vi "Configure Arm Layer Trigger Link.vi"(6 "Enable Output Trigger (F: Disable)":bool, 7 "Arm Output Trigger Line (2: Line2)":i32(ring)=2 items=["Line1"=1, "Line2"=2, "Line3"=3, "Line4"=4, "Line5"=5, "Line6"=6], 8 "error in (no error)":errorcluster, 9 "Arm Input Trigger Line (1: Line1)":i32(ring)=1 items=["Line1"=1, "Line2"=2, "Line3"=3, "Line4"=4, "Line5"=5, "Line6"=6], 10 "Arm Source Bypass (1: Acceptor)":i32(ring)=1 items=["Source", "Acceptor"], 11 "VISA resource name":refnum<visa-resource-name>) -> (0 "error out":errorcluster, 3 "VISA resource name out":refnum<visa-resource-name>)   [LabVIEW 2020, in "Keithley 6517.lvlib"]
doc: "Sets the bypass, input trigger line and output trigger line for the Arm Layer (Arm1) of the trigger model.\n\n<B>Note:</B>\n(1)<B>Models 6517A, 6517B:</B> The trigger model consists of 3 layers, the Arm Layer, the Scan Layer (Arm2), and the Measure Layer (Trigger).\n(2)<B>Model 6514:</B> The trigger model consists of 2 layers: Arm Layer & Measure Layer (Trigger)."
uses:
  <instrlib>/Keithley 6517/Keithley 6517.lvlib
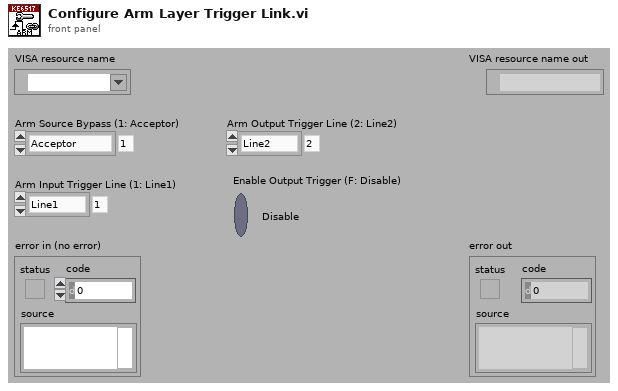
[diagram p1: front panel]
types:
  T1 = typedef "Keithley 6517.lvlib/Extended User Data.ctl" = cluster{"Instrument Model":i32}
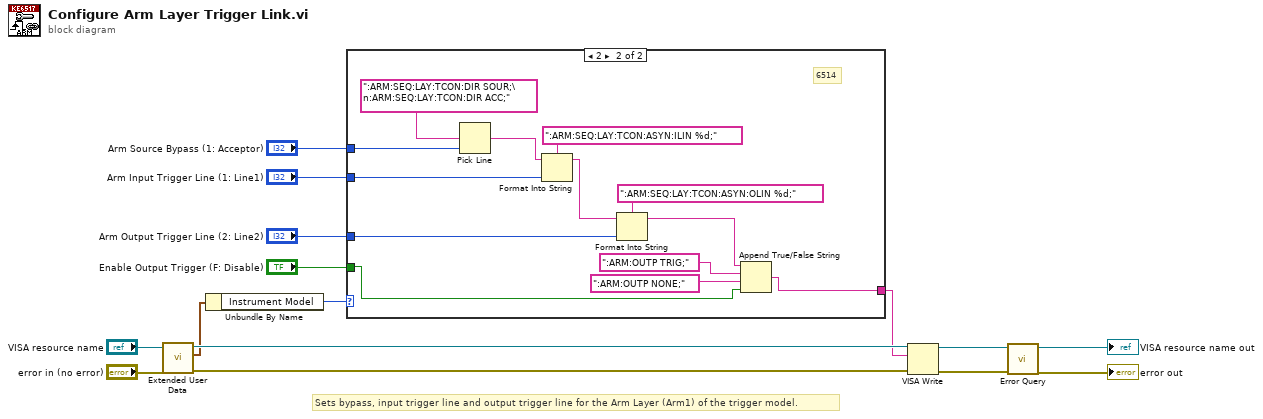
[diagram p0: block diagram]
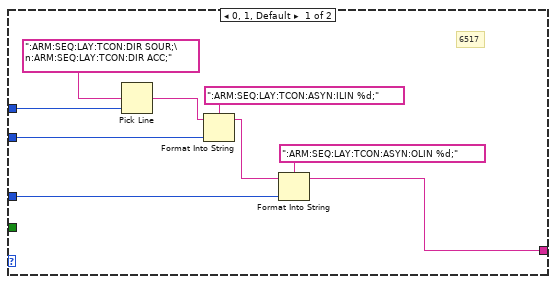
[diagram p2: hidden frame]
diagram:
  # "Sets bypass, input trigger line and output trigger line for the Arm Layer (Arm1) of the trigger model."
  n1 = call <instrlib>:"Extended User Data.vi"("error in (no error)"="error in (no error)", "VISA resource name"="VISA resource name") -> ("error out"=w5:errorcluster, "User Data Out"=w3:T1, "VISA resource name out"=w4:refnum<visa-resource-name>)  [unwired: 7 in]
  n2 = Unbundle By Name(w3) -> ("Instrument Model"=w2:i32)
  n3 = case shown="2" w2 {
    tunnel: "Arm Input Trigger Line (1: Line1)" -> [w23 w36]
    tunnel: "Arm Output Trigger Line (2: Line2)" -> [w20 w33]
    tunnel: "Arm Source Bypass (1: Acceptor)" -> [w18 w31]
    tunnel: "Enable Output Trigger (F: Disable)" -> [_ w27]
    tunnel: [w16 w28] -> w1
    frame 0, 1, Default {
      # "6517"
      n4 = Pick Line(multi-line string=":ARM:SEQ:LAY:TCON:DIR SOUR;\n:ARM:SEQ:LAY:TCON:DIR ACC;", line index=w18) -> (output string=w19:string)  [unwired: 1 in]
      n5 = Format Into String(format string=":ARM:SEQ:LAY:TCON:ASYN:ILIN %d;", initial string=w19, w23) -> (resulting string=w22:string)  [unwired: 1 in, 1 out]
      n6 = Format Into String(format string=":ARM:SEQ:LAY:TCON:ASYN:OLIN %d;", initial string=w22, w20) -> (resulting string=w16:string)  [unwired: 1 in, 1 out]
    }
    frame 2 {
      # "6514"
      n7 = Pick Line(multi-line string=":ARM:SEQ:LAY:TCON:DIR SOUR;\n:ARM:SEQ:LAY:TCON:DIR ACC;", line index=w31) -> (output string=w32:string)  [unwired: 1 in]
      n8 = Format Into String(format string=":ARM:SEQ:LAY:TCON:ASYN:ILIN %d;", initial string=w32, w36) -> (resulting string=w35:string)  [unwired: 1 in, 1 out]
      n9 = Format Into String(format string=":ARM:SEQ:LAY:TCON:ASYN:OLIN %d;", initial string=w35, w33) -> (resulting string=w29:string)  [unwired: 1 in, 1 out]
      n10 = Append True/False String(1:w27, 2:":ARM:OUTP NONE;" ("false string"), 3:":ARM:OUTP TRIG;" ("true string"), 4:w29) -> (0:w28:string)
    }
  }
  n11 = VISA Write(VISA resource name=w4, write buffer=w1, error in (no error)=w5) -> (VISA resource name out=w13:refnum<visa-resource-name>, error out=w12:errorcluster)  [unwired: 1 out]
  n12 = call <instrlib>:"Error Query.vi"("error in (no error)"=w12, "VISA resource name"=w13) -> ("error out"=→"error out":errorcluster, "VISA resource name out"=→"VISA resource name out":refnum<visa-resource-name>)  [unwired: 6 in, 2 out]
